vi "Lidar Initialise.vi"(8 "error in (no error)":errorcluster) -> (0 "error out":errorcluster, 3 "VISA resource name out":refnum<visa-resource-name>)   [LabVIEW 2017]
uses:
  <instrlib>/Hokuyo URG Series/Public/Initialize-cRIO-USB.vi
  <instrlib>/Hokuyo URG Series/Hokuyo URG Series.lvlib
panel:
  in  "Protocol":u32(ring)=2 items=["Convert to Latest", "SCIP 1.1", "SCIP 2.0"]
  in  "ID Query?":bool=TRUE
  in  "Checksum":bool
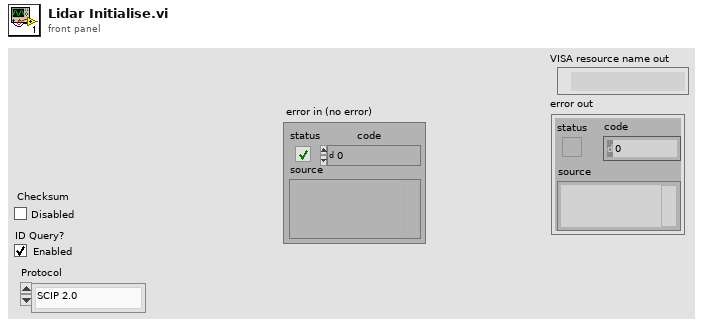
[diagram p1: front panel]
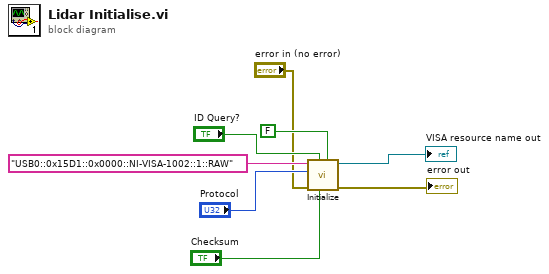
[diagram p0: block diagram]
diagram:
  n1 = call-poly <instrlib>:"Initialize.vi"("Reset? (F: No)"=FALSE ("Reset Instrument (Disabled)"), "Checksum (Disabled)"="Checksum", "ID Query? (Enabled)"="ID Query?", "error in (no error)"="error in (no error)", "Protocol (2: SCIP 2.0)"="Protocol", "VISA resource name"="USB0::0x15D1::0x0000::NI-VISA-1002::1::RAW") -> ("error out"=→"error out":errorcluster, "VISA resource name out"=→"VISA resource name out":refnum<visa-resource-name>)  [unwired: 4 in]
